vi "private_data.set.vi"(10 "private data":refnum<data-value>) -> (3 "Nominal Client":refnum<class "Nominal Client.lvclass">)   [LabVIEW 2020, in "Nominal Client.lvclass"]
uses:
  Nominal Client.lvclass
  private_data.ctl
  <vilib>/addons/_JKI.lib/REST Client/classes/REST Client/REST Client.lvclass
  Nominal Client.lvclass/Nominal Client.ctl
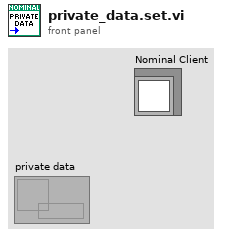
[diagram p1: front panel]
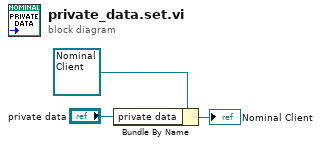
[diagram p0: block diagram]
diagram:
  n1 = Bundle By Name(cluster=refnum<class "Nominal Client.lvclass"> refnum ("Nominal Client"), "private data"="private data") -> (→"Nominal Client":refnum<class "Nominal Client.lvclass">)
